vi "ADIS16460_Open.vi"(8 "error in":errorcluster, 11 "SPI Chip Select":T3=enum."SPI MXP") -> (0 "error out":errorcluster, 3 "ADI IMU Interrupt DevRef":T1={"ADI IMU DevRef"={"DevStatus"={"status"=FALSE, "code"=0, "source"=""}, "Handle"=0, "SPI Bus"=enum."SPI On-Board, CS0", "Device Found"=FALSE, "Device Ready"=FALSE, "Yaw Axis"=enum."Z", "AHRS Algorithm"=enum."Complementary"}, "InterruptRef"={"DevStatus"={"status"=FALSE, "code"=0, "source"=""}, "InterruptIndex"=enum."0"}})   [LabVIEW 2015, in "FRC ADIS16460.lvlib"]
doc: "Initiates communication between an Analog Devices MXP IMU and the RoboRIO."
uses:
  FRC ADIS16460.lvlib
  <vilib>/Rock Robotics/SystemInterfaces/spilib/spi_bus.ctl
  WPI_ADIS16460_InterruptDevRef.ctl
  WPI_ADIS16460_DevRef.ctl
  <vilib>/Rock Robotics/WPI/Interrupt/WPI_InterruptRef.ctl
  <vilib>/Rock Robotics/SystemInterfaces/Interrupt/FPGA_InterruptIndex.ctl
  <vilib>/Rock Robotics/WPI/SPI/WPI_SPIMode.ctl
  <vilib>/Rock Robotics/SystemInterfaces/DIO/FPGA_DIOChannel.ctl
  WPI_IMU_ADIS16460_Registers.ctl
  <vilib>/Rock Robotics/WPI/Counter/WPI_CounterDigitalInputToDigitalSource.vi
  <vilib>/Rock Robotics/SystemInterfaces/CounterEncoderSourceConvertion/FPGA_CounterEncoderSourceConvertionLVSourceTypeToFPGAType.vi
  <vilib>/Rock Robotics/WPI/Interrupt/WPI_InterruptCache.vi
  <vilib>/Rock Robotics/SystemInterfaces/Interrupt/FPGA_InterruptWriteConfiguration.vi
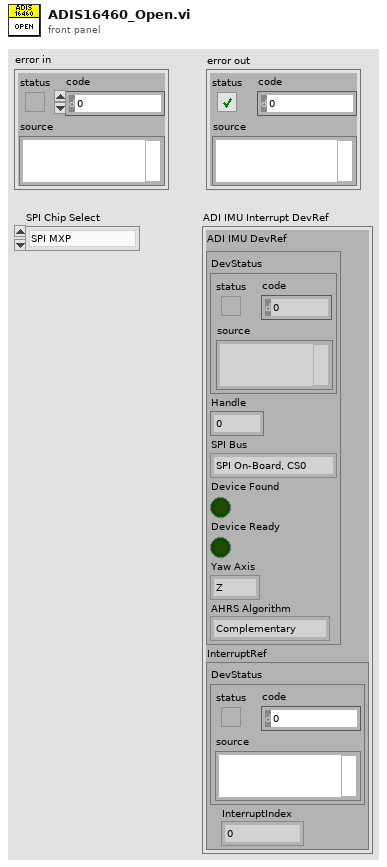
[diagram p1: front panel]
types:
  T1 = typedef "FRC ADIS16460.lvlib/WPI_ADIS16460_InterruptDevRef.ctl" = cluster{"ADI IMU DevRef":T2, "InterruptRef":T4}
  T2 = typedef "FRC ADIS16460.lvlib/WPI_ADIS16460_DevRef.ctl" = cluster{"DevStatus":errorcluster, "Handle":i32, "SPI Bus":T3, "Device Found":bool, "Device Ready":bool, "Yaw Axis":enum16{"X", "Y", "Z"}, "AHRS Algorithm":enum16{"Complementary", "Madgwick"}}
  T3 = typedef "spi_bus.ctl" = enum16{"SPI On-Board, CS0", "SPI On-Board, CS1", "SPI On-Board, CS2", "SPI On-Board, CS3", "SPI MXP", "Invalid"}
  T4 = typedef "WPI_InterruptRef.ctl" = cluster{"DevStatus":errorcluster, "InterruptIndex":T5}
  T5 = typedef "FPGA_InterruptIndex.ctl" = enum8{"0", "1", "2", "3", "4", "5", "6", "7", "Invalid"}
  T6 = typedef "FPGA_DIOChannel.ctl" = enum8{"DIO 0", "DIO 1", "DIO 2", "DIO 3", "DIO 4", "DIO 5", "DIO 6", "DIO 7", "DIO 8", "DIO 9", "DIO MXP 0", "DIO MXP 1", "DIO MXP 2", "DIO MXP 3", "DIO MXP 4", "DIO MXP 5", "DIO MXP 6", "DIO MXP 7", "DIO MXP 8", "DIO MXP 9", "DIO MXP 10", "DIO MXP 11", "DIO MXP 12", "DIO MXP 13", "DIO MXP 14", "DIO MXP 15", "Invalid"}
  T7 = typedef "WPI_SPIMode.ctl" = enum16{"Mode 0 (Clk Idle Low,Sample on Leading)", "Mode 1 (Clk Idle Low,Sample on Trailing)", "Mode 2 (Clk Idle High,Sample on Leading)", "Mode 3 (Clk Idle High,Sample on Trailing)"}
  T8 = typedef "FRC ADIS16460.lvlib/WPI_IMU_ADIS16460_Registers.ctl" = u8
  T9 = typedef "WPI_SPIDevRef.ctl" = cluster{"DevStatus":errorcluster, "Handle":i32, "SPI Bus":T3}
  T10 = typedef "WPI_DigitalInputDevRef.ctl" = cluster{"DevStatus":errorcluster, "DIO Channel":T6}
  T11 = typedef "FPGA_CounterEncoderSourceConvertionLVSourceType.ctl" = cluster{"DevStatus":errorcluster, "AnalogTriggerMode?":bool, "DigitalMode":cluster{"DIO Channel":T12}, "AnalogTriggerMode":cluster{"AnalogTriggerIndex":T13, "OutputType":T14}}
  T12 = typedef "FPGA_DIODigitalSourceChannel.ctl" = enum8{"DIO 0", "DIO 1", "DIO 2", "DIO 3", "DIO 4", "DIO 5", "DIO 6", "DIO 7", "DIO 8", "DIO 9", "DIO MXP 0", "DIO MXP 1", "DIO MXP 2", "DIO MXP 3", "DIO MXP 4", "DIO MXP 5", "DIO MXP 6", "DIO MXP 7", "DIO MXP 8", "DIO MXP 9", "DIO MXP 10", "DIO MXP 11", "DIO MXP 12", "DIO MXP 13", "DIO MXP 14", "DIO MXP 15", "Disabled"}
  T13 = typedef "FPGA_AnalogTriggerIndex.ctl" = enum8{"Trig 0", "Trig 1", "Trig 2", "Trig 3", "Trig 4", "Trig 5", "Trig 6", "Trig 7", "Invalid"}
  T14 = typedef "FPGA_AnalogTriggerOutType.ctl" = enum16{"InWindow", "TriggerState", "Rising", "Falling"}
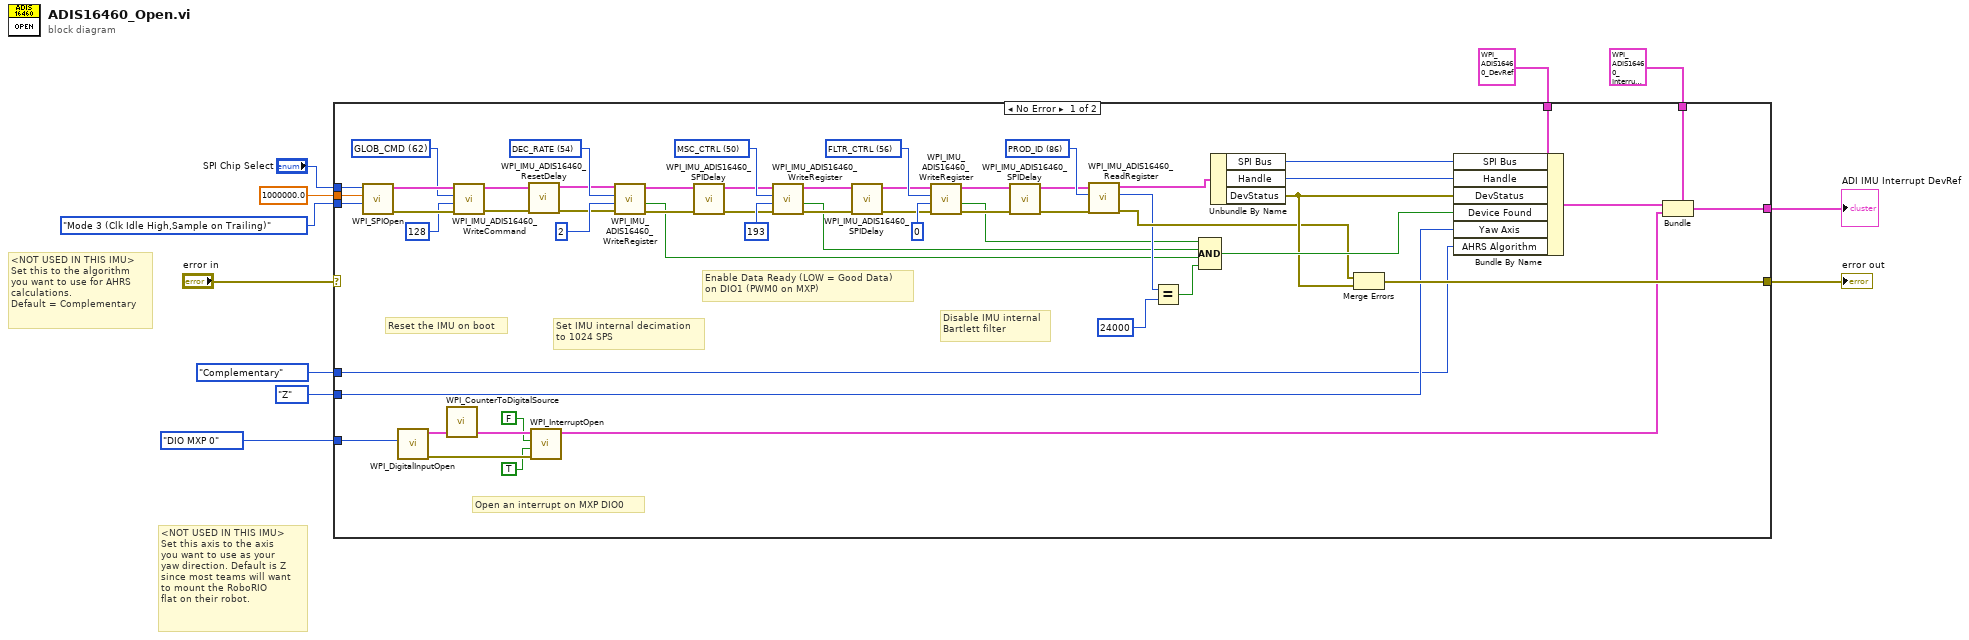
[diagram p0: block diagram]
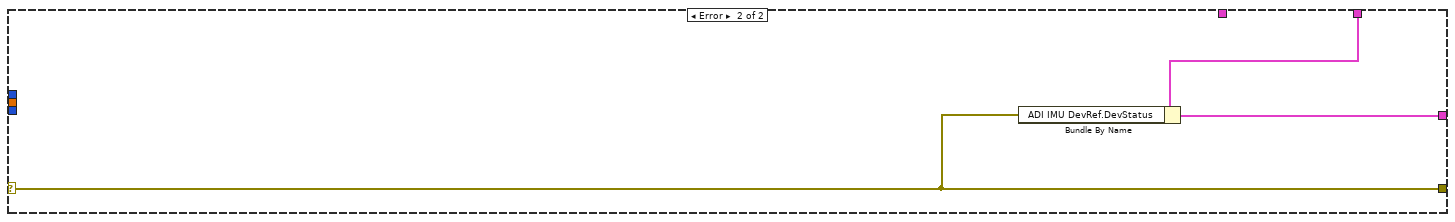
[diagram p2: hidden frame]
diagram:
  # "<NOT USED IN THIS IMU>\nSet this to the algorithm\nyou want to use for AHRS\ncalculations. \nDefault = Complementary"
  # "<NOT USED IN THIS IMU>\nSet this axis to the axis\nyou want to use as your\nyaw direction. Default is Z\nsince most teams will want \nto mount the RoboRIO\nflat on their robot."
  n1 = case shown="No Error" "error in" {
    selector: "error in" -> [_ w69]
    tunnel: "SPI Chip Select" -> [w67 _]
    tunnel: 1000000.0 ("Clock Rate (Hz)") -> [w66 _]
    tunnel: WPI_SPIMode."Mode 3 (Clk Idle High,Sample on Trailing)" ("Mode (3)") -> [w65 _]
    tunnel: [w58 w69] -> w7
    tunnel: T2 {"DevStatus"={"status"=FALSE, "code"=0, "source"=""}, "Handle"=0, "SPI Bus"=enum."SPI On-Board, CS0", "Device Found"=FALSE, "Device Ready"=FALSE, "Yaw Axis"=enum."Z", "AHRS Algorithm"=enum."Complementary"} ("SimpleGyroDevRef 2") -> [w64 _]
    tunnel: [w49 w68] -> w1
    tunnel: T1 {"ADI IMU DevRef"={"DevStatus"={"status"=FALSE, "code"=0, "source"=""}, "Handle"=0, "SPI Bus"=enum."SPI On-Board, CS0", "Device Found"=FALSE, "Device Ready"=FALSE, "Yaw Axis"=enum."Z", "AHRS Algorithm"=enum."Complementary"}, "InterruptRef"={"DevStatus"={"status"=FALSE, "code"=0, "source"=""}, "InterruptIndex"=enum."0"}} ("output cluster") -> [w48 w70]
    tunnel: FPGA_DIOChannel."DIO MXP 0" ("DIO Channel") -> [w47 _]
    tunnel: enum16{"X", "Y", "Z"}."Z" ("Yaw Axis") -> [w41 _]
    tunnel: enum16{"Complementary", "Madgwick"}."Complementary" ("AHRS Algorithm") -> [w40 _]
    frame No Error {
      w13 = T8 62 items=["PROD_ID"=86, "GLOB_CMD"=62, "DEC_RATE"=54, "FLTR_CTRL"=56, "MSC_CTRL"=50] ("ADIS16448 Register")
      w36 = T8 56 items=["PROD_ID"=86, "GLOB_CMD"=62, "DEC_RATE"=54, "FLTR_CTRL"=56, "MSC_CTRL"=50] ("ADIS16448 Register")
      w37 = T8 50 items=["PROD_ID"=86, "GLOB_CMD"=62, "DEC_RATE"=54, "FLTR_CTRL"=56, "MSC_CTRL"=50] ("ADIS16448 Register")
      w38 = T8 54 items=["PROD_ID"=86, "GLOB_CMD"=62, "DEC_RATE"=54, "FLTR_CTRL"=56, "MSC_CTRL"=50] ("ADIS16448 Register")
      w39 = T8 86 items=["PROD_ID"=86, "GLOB_CMD"=62, "DEC_RATE"=54, "FLTR_CTRL"=56, "MSC_CTRL"=50] ("ADIS16448 Register")
      # "Reset the IMU on boot"
      # "Open an interrupt on MXP DIO0"
      # "Disable IMU internal\nBartlett filter"
      # "Enable Data Ready (LOW = Good Data) \non DIO1 (PWM0 on MXP)"
      # "Set IMU internal decimation\nto 1024 SPS"
      n2 = call <vilib>:"WPI_SPIOpen.vi"("Mode (3)"=w65, "Clock Rate (Hz)"=w66, "SPI Bus"=w67) -> ("error out"=w18:errorcluster, "SPIDevRef"=w19:T9)  [unwired: 7 in]
      n3 = call <vilib>:"WPI_DigitalInputOpen.vi"("DIO Channel"=w47) -> ("error out"=w54:errorcluster, "DigitalInputDevRef"=w56:T10)  [unwired: 9 in]
      n4 = call-poly <vilib>:"WPI_CounterToDigitalSource.vi"("DigitalInputDevRef"=w56) -> ("Digital Source"=w55:T11)  [unwired: 6 in]
      n5 = call "WPI_IMU_ADIS16460_WriteCommand.vi"("error in (no error)"=w18, "Data"=u16 128, "ADIS16460 Register"=w13, "SPIDevRef in"=w19) -> ("error out"=w17:errorcluster, "SPIDevRef out"=w16:T9)  [unwired: 6 in]
      n6 = call "WPI_IMU_ADIS16460_ResetDelay.vi"("error in"=w17, "SPIDevRef in"=w16) -> ("error out"=w14:errorcluster, "SPIDevRef out"=w15:T9)  [unwired: 8 in]
      n7 = call <vilib>:"WPI_InterruptOpen.vi"("error in (no error)"=w54, "Falling Edge"=TRUE, "Rising Edge"=FALSE, "Source"=w55) -> ("InterruptRef"=w51:T4)  [unwired: 6 in, 1 out]
      n8 = call "WPI_IMU_ADIS16460_WriteRegister.vi"("error in (no error)"=w14, "Data"=u16 2, "ADIS16460 Register"=w38, "SPIDevRef in"=w15) -> ("error out"=w35:errorcluster, "Write OK?"=w23:bool, "SPIDevRef out"=w34:T9)  [unwired: 4 in, 1 out]
      n9 = call "WPI_IMU_ADIS16460_SPIDelay.vi"("error in"=w35, "SPIDevRef in"=w34) -> ("error out"=w32:errorcluster, "SPIDevRef out"=w33:T9)  [unwired: 8 in]
      n10 = call "WPI_IMU_ADIS16460_WriteRegister.vi"("error in (no error)"=w32, "Data"=u16 193, "ADIS16460 Register"=w37, "SPIDevRef in"=w33) -> ("error out"=w30:errorcluster, "Write OK?"=w22:bool, "SPIDevRef out"=w31:T9)  [unwired: 4 in, 1 out]
      n11 = call "WPI_IMU_ADIS16460_SPIDelay.vi"("error in"=w30, "SPIDevRef in"=w31) -> ("error out"=w28:errorcluster, "SPIDevRef out"=w29:T9)  [unwired: 8 in]
      n12 = call "WPI_IMU_ADIS16460_WriteRegister.vi"("error in (no error)"=w28, "Data"=u16 0, "ADIS16460 Register"=w36, "SPIDevRef in"=w29) -> ("error out"=w27:errorcluster, "Write OK?"=w21:bool, "SPIDevRef out"=w26:T9)  [unwired: 4 in, 1 out]
      n13 = call "WPI_IMU_ADIS16460_SPIDelay.vi"("error in"=w27, "SPIDevRef in"=w26) -> ("error out"=w24:errorcluster, "SPIDevRef out"=w25:T9)  [unwired: 8 in]
      n14 = call "WPI_IMU_ADIS16460_ReadRegister.vi"("error in (no error)"=w24, "ADIS16460 Register"=w39, "SPIDevRef in"=w25) -> ("error out"=w45:errorcluster, "Register Value"=w44:u16, "SPIDevRef out"=w46:T9)  [unwired: 6 in]
      n15 = Equal?(x=w44, y=u16 24000) -> (x = y?=w20:bool)
      n16 = Compound Arithmetic op=AND(w21, w22, w23, w20) -> (w60:bool)
      n17 = Unbundle By Name(w46) -> ("SPI Bus"=w63:T3, "Handle"=w62:i32, "DevStatus"=w59:errorcluster)
      n18 = Merge Errors(w45, w59) -> (w58:errorcluster)
      n19 = Bundle By Name(cluster=w64, "SPI Bus"=w63, "Handle"=w62, "DevStatus"=w59, "Device Found"=w60, "Yaw Axis"=w41, "AHRS Algorithm"=w40) -> (w50:T2)
      n20 = Bundle(cluster=w48, "ADI IMU DevRef"=w50, "InterruptRef"=w51) -> (w49:T1)
    }
    frame Error {
      n21 = Bundle By Name(cluster=w70, "ADI IMU DevRef.DevStatus"=w69) -> (w68:T1)
    }
  }
  "error out" <- w7
  "ADI IMU Interrupt DevRef" <- w1
